vi "Constants.vi"() -> ()   [LabVIEW 2020, in "PXI-2510 Shared.lvlib"]
doc: "Use this Global VI to access the GUIDs assigned to the page resources of the Custom Device."
uses:
  PXI-2510 Shared.lvlib
panel:
  in  "Tab Control":enum32{"GUIDs", "Constants", "Properties"}(tab)
  in  "Disable PXI-2510 GUID":string="865bd9fa-a155-4566-879d-0834230785a3"
  in  "PXI-2510 Channel Page":string="10cc04ef-3542-46d8-a2d9-8d0ca505f877"
  in  "PXI-2510 Fault Bus Page":string="1ca83dac-4ca4-4634-b3f6-f8ba7047293d"
  in  "PXI-2510":string="1d96ea35-2726-401d-a052-f61bcf1a45df"
  in  "Fault Channel Description":string="The \"Name (Alias)\" for each channel may be changed. The \"Hardware Channel #\" cannot be changed by the user, and represents the actual Fault Channel being controller.\n\nThe Fault Default Value sets the default state for the channel."
  in  "Fault Bus Description":string="The Fault Bus has 6 different options: Default, Input 0, Input 1, Input 2, Input 3, and Main Bus Only.\n\nDefault: Does not make a call to the driver.\n\nInput 0,1,2,3: Close thier respective lines so that both the Main Bus and the Input Line is connected to the Fault Bus\n\nMain Bus Only: Disconnects Inputs 0,1,2, and 3 so that the Main Bus line is the only one connected to the Fault Bus"
  in  "Fault Bus Input Selector":string="Fault Bus Input Selector"
  in  "Channel Fault":string="Channel Fault"
  in  "Hardware Device Name":string="Hardware Device Name"
  in  "FIU Description":string="This is a Custom Device for the PXI-2510 FIU."
  in  "FIU Channel #":string="FIU Channel #"
  in  "Compiled.Settings":string="Compiled.Settings"
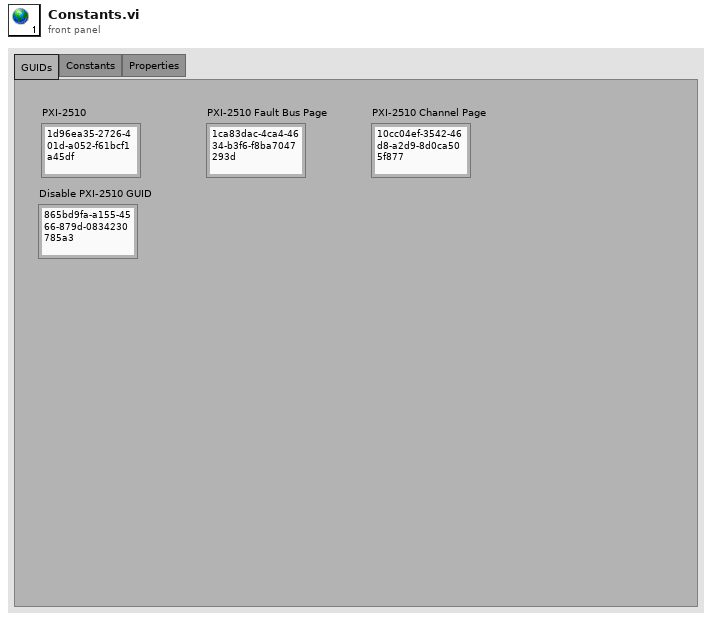
[diagram p1: front panel]
diagram:
